vi "MALTCON inc miant counter.vi"() -> ()   [LabVIEW 2018]
uses:
  <instrlib>/AltonTech MALT/AltonTech MALT200817.lvlib
panel:
  in  "Address":i32=1
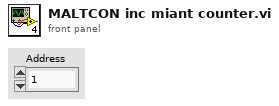
[diagram p1: front panel]
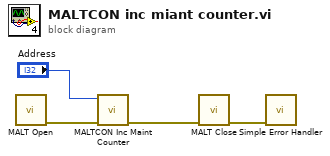
[diagram p0: block diagram]
diagram:
  n1 = call <instrlib>:"MALT Open.vi"() -> ("error out"=w3:errorcluster)  [unwired: 10 in, 1 out]
  n2 = call <instrlib>:"MALTCON Inc Maint Counter.vi"("error in"=w3, "Address"="Address") -> ("error out"=w4:errorcluster)  [unwired: 9 in]
  n3 = call <instrlib>:"MALT Close.vi"("error in"=w4) -> ("error out"=w2:errorcluster)  [unwired: 10 in]
  n4 = call <vilib>:"Simple Error Handler.vi"("error in (no error)"=w2) -> ()  [unwired: 4 in, 5 out]
